vi "convert_table.vi"(9 "Table Doubles":dbl[][](array[numeric])) -> (1 "Table Strings":string[][](array[string]))   [LabVIEW 2021, in "Certification.lvlib"]
uses:
  Certification.lvlib
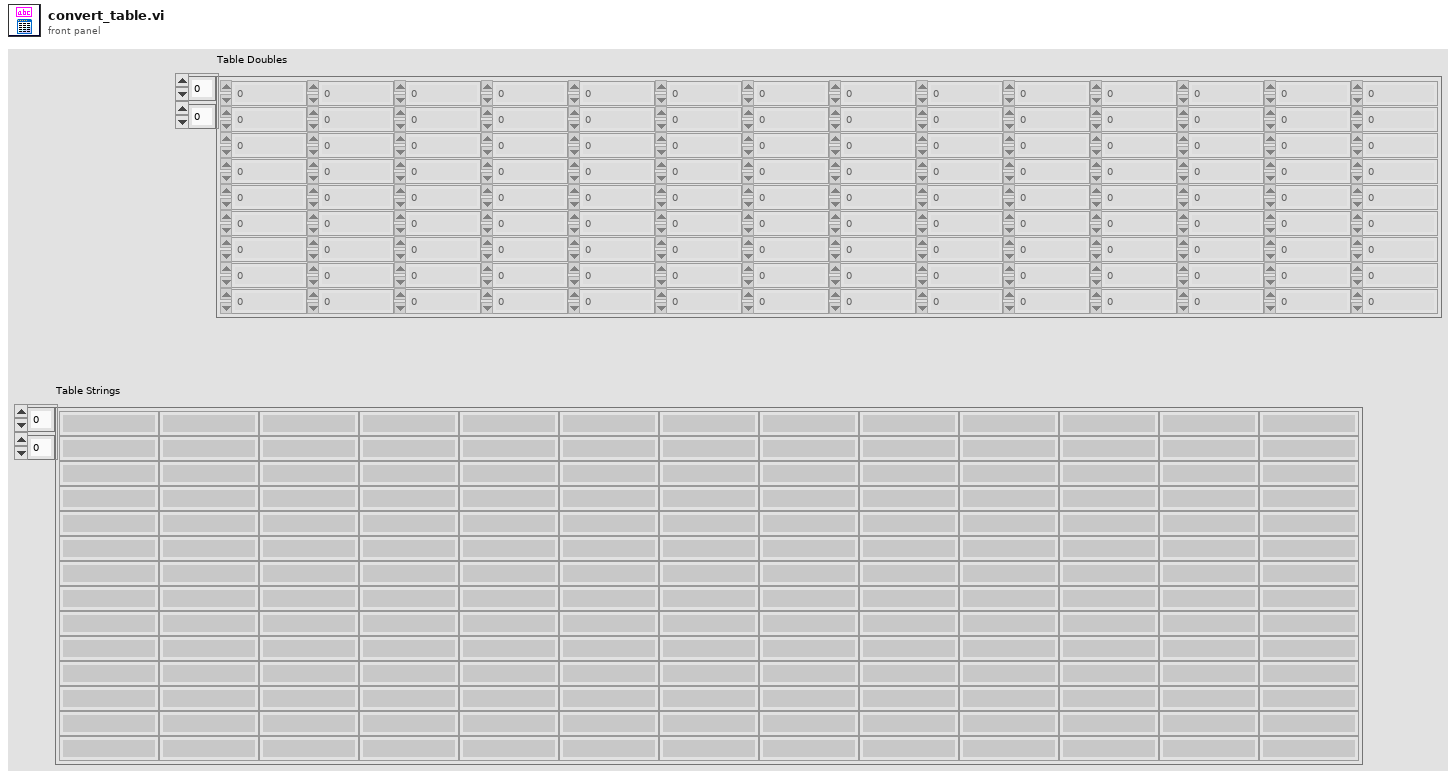
[diagram p1: front panel]
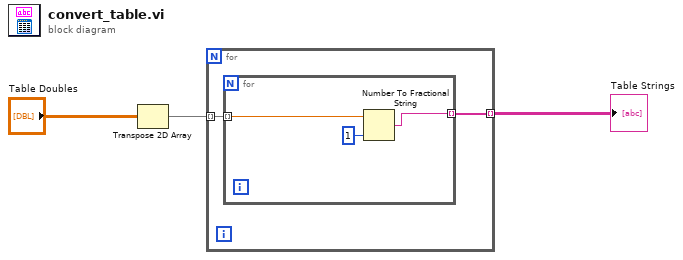
[diagram p0: block diagram]
diagram:
  n1 = Transpose 2D Array(2D array="Table Doubles") -> (transposed array=w2:dbl[][])
  n2 = for {
    tunnel: w2 -> [w5] mode=indexing
    tunnel: [w4] -> w3 mode=indexing
    n3 = for {
      tunnel: w5 -> [w6] mode=indexing
      tunnel: [w7] -> w4 mode=indexing
      n4 = Number To Fractional String(number=w6, precision (6)=i16 1) -> (F-format string=w7:string)  [unwired: 2 in]
    }
  }
  "Table Strings" <- w3
